vi "Parse (Euler Angles).vi"(7 "Message In":string) -> (6 "Roll":sgl, 8 "Pitch":sgl, 10 "Yaw":sgl, 15 "Timer":u32)   [LabVIEW 2012, in "MicroStrain 3DM-GXx.lvlib"]
doc: "Parse the data from the 0xCE message into Roll (rad), Pitch (rad), and Yaw (rad)."
uses:
  <instrlib>/MicroStrain 3DM-GXx/MicroStrain 3DM-GXx.lvlib
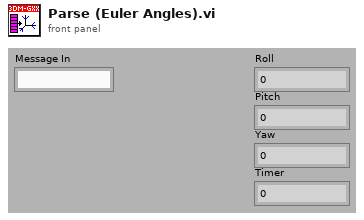
[diagram p1: front panel]
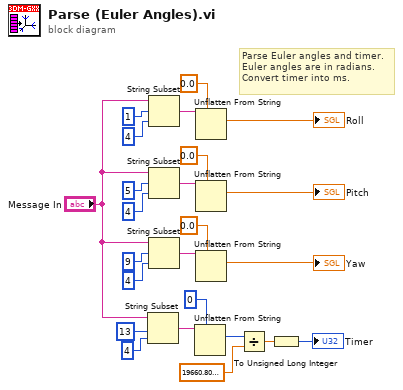
[diagram p0: block diagram]
diagram:
  # "Parse Euler angles and timer.\nEuler angles are in radians.\nConvert timer into ms."
  n1 = String Subset(string="Message In", offset (0)=13, length (rest)=4 ("length (rest)")) -> (substring=w9:string)
  n2 = String Subset(string="Message In", offset (0)=1, length (rest)=4 ("length (rest)")) -> (substring=w22:string)
  n3 = String Subset(string="Message In", offset (0)=5, length (rest)=4 ("length (rest)")) -> (substring=w19:string)
  n4 = String Subset(string="Message In", offset (0)=9, length (rest)=4 ("length (rest)")) -> (substring=w14:string)
  n5 = Unflatten From String(type=u32 0, binary string=w9) -> (value=w8:u32)  [unwired: 3 in, 2 out]
  n6 = Unflatten From String(type=sgl 0.0, binary string=w22) -> (value=→"Roll":sgl)  [unwired: 3 in, 2 out]
  n7 = Unflatten From String(type=sgl 0.0, binary string=w19) -> (value=→"Pitch":sgl)  [unwired: 3 in, 2 out]
  n8 = Unflatten From String(type=sgl 0.0, binary string=w14) -> (value=→"Yaw":sgl)  [unwired: 3 in, 2 out]
  n9 = Divide(x=w8, y=sgl 19660.8) -> (x/y=w6:sgl)
  n10 = To Unsigned Long Integer(number=w6) -> (unsigned 32bit integer=→"Timer":u32)
